vi "H5Iget_ref.vi"(6 "error in (no error)":errorcluster, 9 "HDF5 Ref":T1) -> (0 "error out":errorcluster, 2 "HDF5 File Ref":i32, 3 "HDF5 Ref out":T1)   [LabVIEW 2017]
doc: "Retrieves the reference count for an object."
uses:
  <vilib>/UPVI/lvhdf5/library.llb/HDF5 Ref.ctl
  <vilib>/UPVI/lvhdf5/hdf5.dll
panel:
  # "LVHDF5 Toolkit\nCopyright (c) 2005-2013 by Jason D. Sommerville\nCopyright (c) 2014 by UPVI, LLC.\n\nThis use and distribution of this file is governed by the terms found in \nLICENSE.txt distributed with this toolkit and installed at\n <user.lib>\\_lvhdf5\\LICENSE.txt"
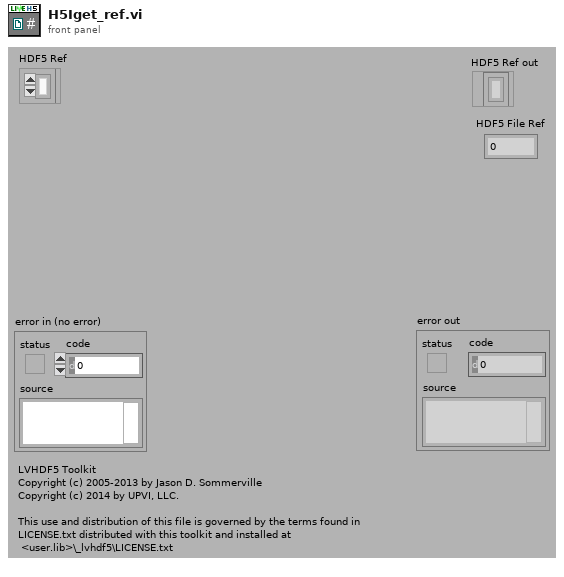
[diagram p1: front panel]
types:
  T1 = typedef "HDF5 Ref.ctl" = refnum<k1>
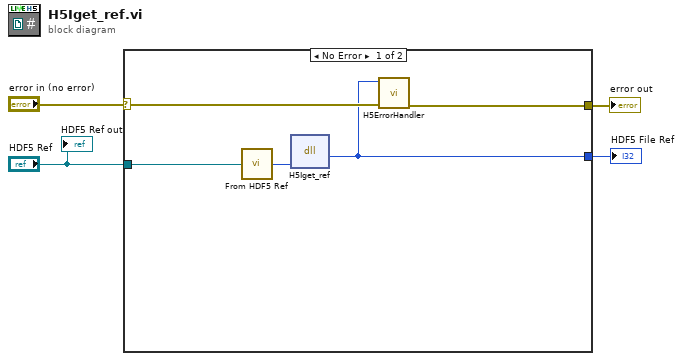
[diagram p0: block diagram]
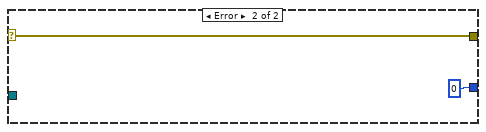
[diagram p2: hidden frame]
diagram:
  n1 = case shown="No Error" "error in (no error)" {
    selector: "error in (no error)" -> [w7 w11]
    tunnel: [w6 w11] -> w2
    tunnel: "HDF5 Ref" -> [w9 _]
    tunnel: [w5 0] -> w1
    frame No Error {
      n2 = call <vilib>:"From HDF5 Ref.vi"("HDF5 Ref"=w9) -> ("I32"=w8:i32)
      n3 = dll-call lib="C:/Program Files/National Instruments/LabVIEW 2017/vi.lib/UPVI/lvhdf5/hdf5.dll" fn="H5Iget_ref"("attr_id"=w8) -> (w5:i32)  [unwired: 4 in, 2 out]
      n4 = call <vilib>:"H5ErrorHandler.vi"("error in (no error)"=w7, "herr_t"=w5) -> ("error out"=w6:errorcluster)  [unwired: 3 in, 4 out]
    }
    frame Error {
    }
  }
  "error out" <- w2
  "HDF5 File Ref" <- w1
  "HDF5 Ref out" <- "HDF5 Ref"
